vi "test-Rect-Region-Constraint-Test1.vi"(8 "error in (no error)":errorcluster) -> (0 "error out":errorcluster, 3 "All tests passed":bool)   [LabVIEW 2019]
uses:
  <vilib>/Rock Robotics/WPI/ThirdParty/JAS_Junk/TrajLib/TypeDef/TRAJ_CONSTRAINT_RECT_REGION.ctl
  <vilib>/Rock Robotics/WPI/ThirdParty/JAS_Junk/TrajLib/TRANSLATION2D.ctl
  <vilib>/Rock Robotics/WPI/ThirdParty/JAS_Junk/TrajLib/Enum/TRAJ_CONSTRAINT_TYPES_ENUM.ctl
  <vilib>/Rock Robotics/WPI/ThirdParty/JAS_Junk/TrajLib/TRAJECTORY.ctl
  <vilib>/Rock Robotics/WPI/ThirdParty/JAS_Junk/TrajLib/TRAJ_STATE.ctl
  <vilib>/Rock Robotics/WPI/ThirdParty/JAS_Junk/TrajLib/POSE2D.ctl
  <vilib>/Rock Robotics/WPI/ThirdParty/JAS_Junk/TrajLib/ROTATION2D.ctl
  <vilib>/Rock Robotics/WPI/ThirdParty/JAS_Junk/TrajLib/TRAJ_CONFIG.ctl
  <vilib>/Rock Robotics/WPI/ThirdParty/JAS_Junk/TrajLib/VI/TrajConstraint_GetType.vi
  <vilib>/Utility/Data Type/Get Type Information.vi
  <vilib>/Rock Robotics/WPI/ThirdParty/JAS_Junk/TrajLib/Trajectory_Library.lvlib
panel:
  out "Was in region":bool
  out "Didnt Exceed Inside":bool
  out "Exceeded outside":bool
  out "outTRAJECTORY_CONFIG":T1 {"End Velocity" format="%20.4f"; "StartVelocity" format="%20.4f"; "Max Acceleration" format="%20.4f"; "MaxVelocity" format="%20.4f"}
  out "PoseInRegion":bool
  out "error out 2":errorcluster
  out "TRAJECTORY":T2 {"States"."POSE"."ROTATION"."SIN" format="%13.4f"; "States"."POSE"."ROTATION"."COS" format="%13.4f"; "States"."POSE"."ROTATION"."VALUE" format="%13.4f"; "States"."POSE"."TRANSLATION"."Y" format="%14.3f"; "States"."POSE"."TRANSLATION"."X" format="%14.3f"; "TotalTImeSecs" format="%20.3f"}
  out "RECT_REGION_CONSTRAINT":T7={"BottomLeftPoint"={"X"=0.0, "Y"=0.0}, "TopRightPoint"={"X"=0.0, "Y"=0.0}, "Constraint"=variant, "Constraint Type"=enum."DIFF DRIVE KINEMATICS"} {"TopRightPoint"."Y" format="%14.3f"; "TopRightPoint"."X" format="%14.3f"; "BottomLeftPoint"."Y" format="%14.3f"; "BottomLeftPoint"."X" format="%14.3f"}
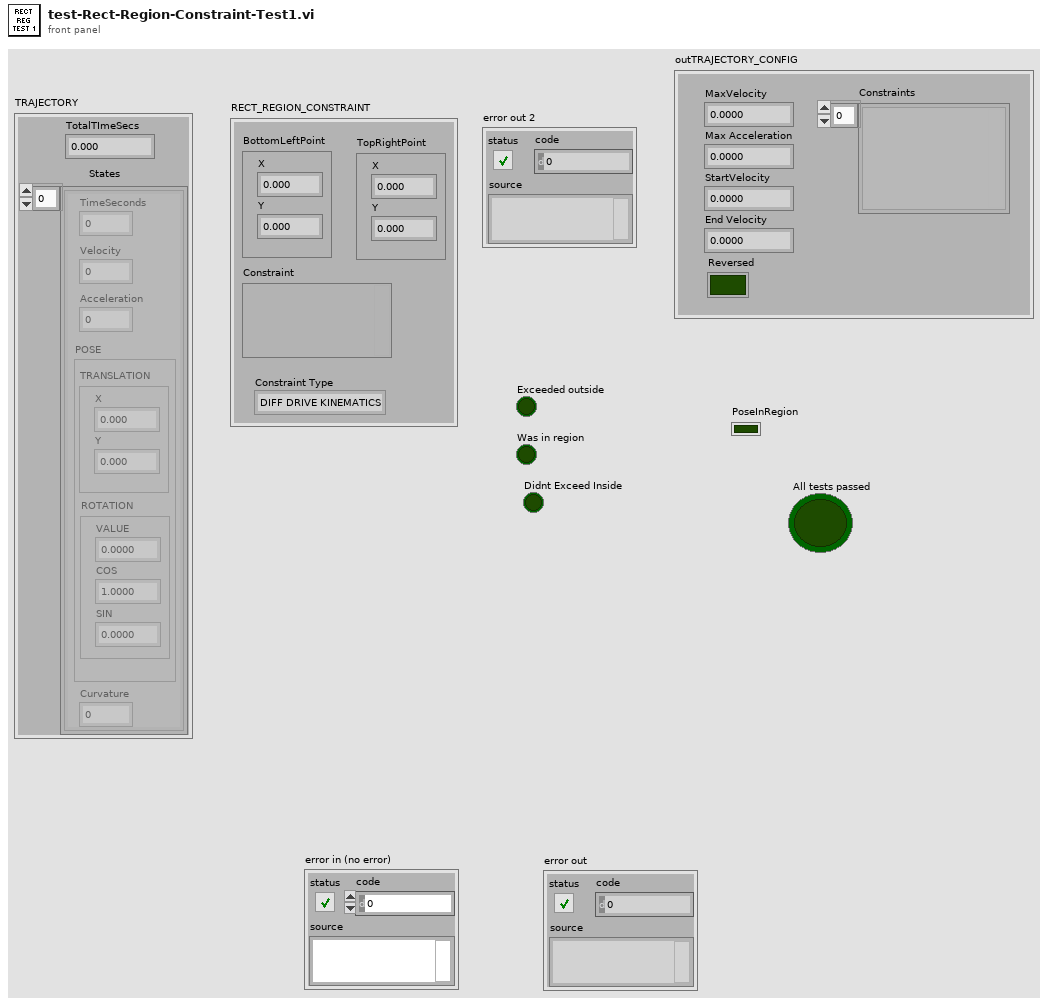
[diagram p1: front panel]
types:
  T1 = typedef "Trajectory_Library.lvlib/TRAJ_CONFIG.ctl" = cluster{"MaxVelocity":dbl, "Max Acceleration":dbl, "StartVelocity":dbl, "End Velocity":dbl, "Reversed":bool, "Constraints":variant[]}
  T2 = typedef "Trajectory_Library.lvlib/TRAJECTORY.ctl" = cluster{"TotalTImeSecs":dbl, "States":T3[]}
  T3 = typedef "Trajectory_Library.lvlib/TRAJ_STATE.ctl" = cluster{"TimeSeconds":dbl, "Velocity":dbl, "Acceleration":dbl, "POSE":T4, "Curvature":dbl}
  T4 = typedef "Trajectory_Library.lvlib/POSE2D.ctl" = cluster{"TRANSLATION":T5, "ROTATION":T6}
  T5 = typedef "Trajectory_Library.lvlib/TRANSLATION2D.ctl" = cluster{"X":dbl, "Y":dbl}
  T6 = typedef "Trajectory_Library.lvlib/ROTATION2D.ctl" = cluster{"VALUE":dbl, "COS":dbl, "SIN":dbl}
  T7 = typedef "Trajectory_Library.lvlib/TRAJ_CONSTRAINT_RECT_REGION.ctl" = cluster{"BottomLeftPoint":T5, "TopRightPoint":T5, "Constraint":variant, "Constraint Type":T8}
  T8 = typedef "Trajectory_Library.lvlib/TRAJ_CONSTRAINT_TYPES_ENUM.ctl" = enum16{"UNDEFINED", "DIFF DRIVE KINEMATICS", "DIFF DRIVE VOLTAGE", "CENTRIPITAL ACCEL", "MECA DRIVE KINEMATICS", "SWERVE DRIVE KINEMATICS", "MAXIMUM VELOCITY"}
  T9 = typedef "Trajectory_Library.lvlib/TRAJ_CONSTRAINT_MAX_VELOCITY.ctl" = cluster{"Max Velocity":dbl, "IM UNIQUE":bool}
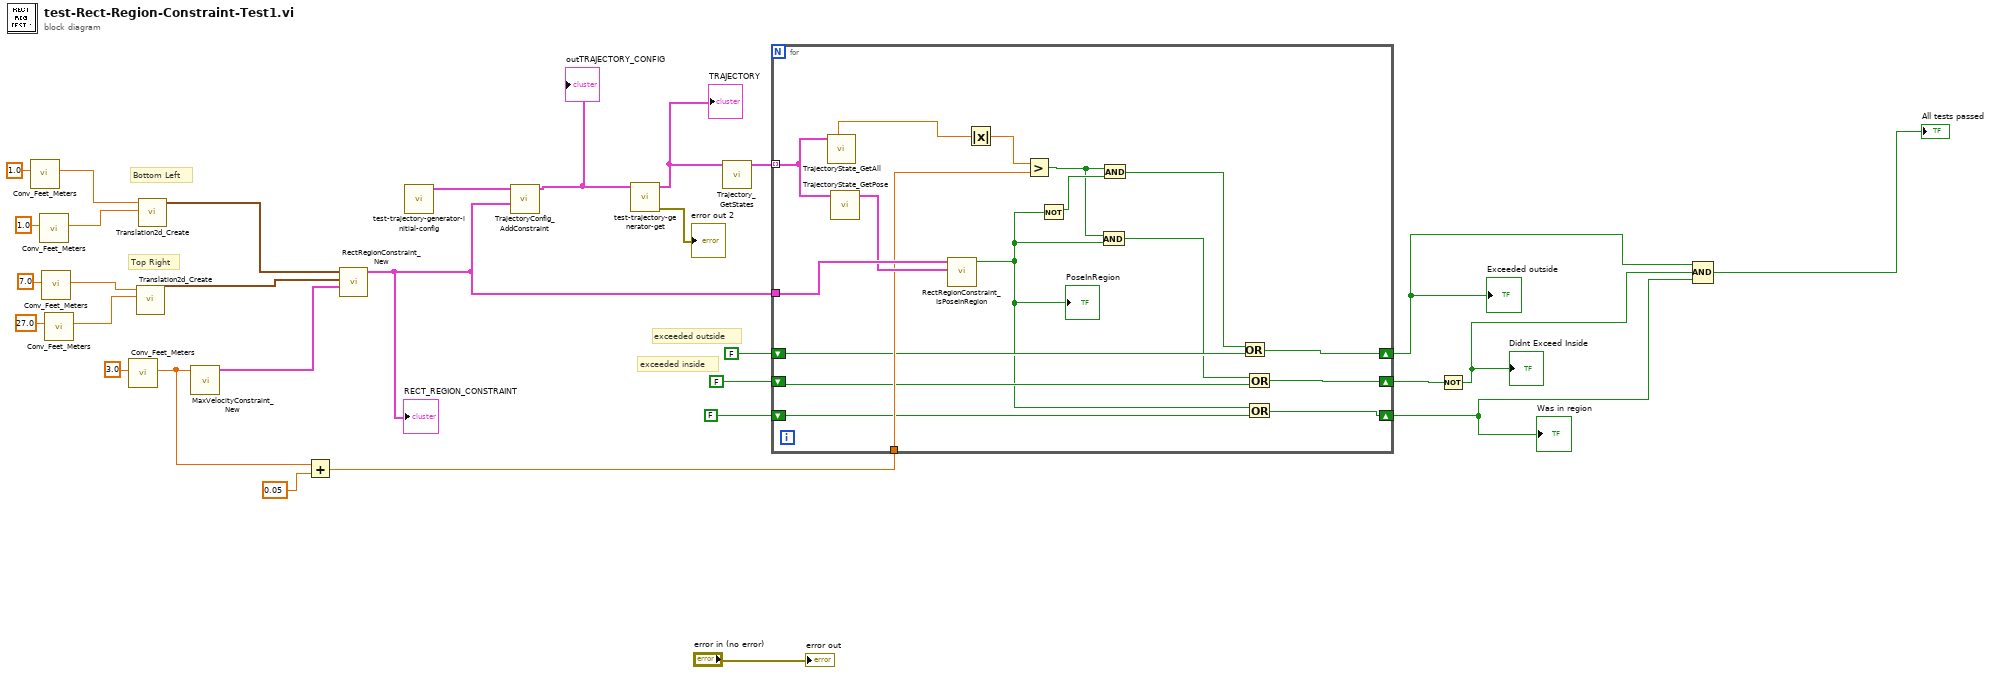
[diagram p0: block diagram]
diagram:
  # "exceeded inside"
  # "exceeded outside"
  # "Top Right"
  # "Bottom Left"
  n1 = call <vilib>:"Conv_Feet_Meters.vi"("Feet"=1.0) -> ("Meters"=w21:dbl)  [unwired: 10 in]
  n2 = call <vilib>:"Conv_Feet_Meters.vi"("Feet"=1.0) -> ("Meters"=w20:dbl)  [unwired: 10 in]
  n3 = call <vilib>:"Conv_Feet_Meters.vi"("Feet"=7.0) -> ("Meters"=w19:dbl)  [unwired: 10 in]
  n4 = call <vilib>:"Conv_Feet_Meters.vi"("Feet"=27.0) -> ("Meters"=w18:dbl)  [unwired: 10 in]
  n5 = call <vilib>:"Conv_Feet_Meters.vi"("Feet"=3.0) -> ("Meters"=w10:dbl)  [unwired: 10 in]
  n6 = call <vilib>:"Translation2d_Create.vi"("Y"=w18, "X"=w19) -> ("TRANSLATION"=w27:T5)  [unwired: 9 in]
  n7 = call <vilib>:"Translation2d_Create.vi"("Y"=w20, "X"=w21) -> ("TRANSLATION"=w28:T5)  [unwired: 9 in]
  n8 = call <vilib>:"MaxVelocityConstraint_New.vi"("Maximum Velocity"=w10) -> ("MAX_VELOCITY_CONSTRAINT"=w26:T9)  [unwired: 10 in]
  n9 = Add(x=w10, y=0.05) -> (x+y=w8:dbl)
  n10 = call <vilib>:"RectRegionConstraint_New.vi"("Constraint Data Cluster"=w26, "TopRightPoint"=w27, "BottomLeftPoint"=w28) -> ("RECT_REGION_CONSTRAINT"=w12:T7)  [unwired: 8 in]
  "RECT_REGION_CONSTRAINT" <- w12
  n11 = call "test-trajectory-generator-initial-config.vi"() -> ("traj_config"=w17:T1)  [unwired: 11 in]
  n12 = call <vilib>:"TrajectoryConfig_AddConstraint.vi"("Constraint"=w12, "inTRAJECTORY_CONFIG"=w17) -> ("outTRAJECTORY_CONFIG"=w16:T1)  [unwired: 9 in]
  "outTRAJECTORY_CONFIG" <- w16
  n13 = call "test-trajectory-generator-get.vi"("traj_config"=w16) -> ("error out"=→"error out 2":errorcluster, "TRAJECTORY"=w14:T2)  [unwired: 8 in, 1 out]
  "TRAJECTORY" <- w14
  n14 = call <vilib>:"Trajectory_GetStates.vi"("TRAJECTORY"=w14) -> ("States"=w13:T3[])  [unwired: 10 in]
  n15 = for {
    tunnel: w13 -> [w46] mode=indexing
    tunnel: w12 -> [w47]
    shift-right: [w44] -> w5
    shift-left: FALSE -> [w38]
    tunnel: w8 -> [w41]
    shift-right: [w34] -> w4
    shift-left: FALSE -> [w35]
    shift-right: [w31] -> w2
    shift-left: FALSE -> [w32]
    n16 = call <vilib>:"TrajectoryState_GetAll.vi"("TRAJ_STATE"=w46) -> ("Velocity"=w43:dbl)  [unwired: 4 in, 6 out]
    n17 = call <vilib>:"TrajectoryState_GetPose.vi"("TRAJ_STATE"=w46) -> ("TrajStatePose"=w45:T4)  [unwired: 10 in]
    n18 = call <vilib>:"RectRegionConstraint_IsPoseInRegion.vi"("statePose"=w45, "RECT_REGION_CONSTRAINT"=w47) -> ("PoseInRegion"=w33:bool)  [unwired: 9 in]
    "PoseInRegion" <- w33
    n19 = Absolute Value(x=w43) -> (abs(x)=w42:dbl)
    n20 = Greater?(x=w42, y=w41) -> (0:w37:bool)
    n21 = Not(x=w33) -> (.not. x?=w40:bool)
    n22 = And(x=w37, y=w33) -> (x .and. y?=w36:bool)
    n23 = And(x=w37, y=w40) -> (x .and. y?=w39:bool)
    n24 = Or(x=w39, y=w38) -> (x .or. y?=w44:bool)
    n25 = Or(x=w36, y=w35) -> (x .or. y?=w34:bool)
    n26 = Or(x=w33, y=w32) -> (x .or. y?=w31:bool)
  }
  "Exceeded outside" <- w5
  "Was in region" <- w2
  n27 = Not(x=w4) -> (.not. x?=w3:bool)
  "Didnt Exceed Inside" <- w3
  n28 = Compound Arithmetic op=AND(w5, w3, w2) -> (→"All tests passed":bool)
  "error out" <- "error in (no error)"
